vi "Subscribe (Async).vi"(9 "Topic":string, 10 "error in (no error)":errorcluster, 11 "WAMP Client in":refnum<class "WAMP Client.lvclass">) -> (1 "Request Result Event":refnum<user-event>, 2 "error out":errorcluster, 3 "WAMP Client out":refnum<class "WAMP Client.lvclass">)   [LabVIEW 2020, in "wamplv.lvlib" / "WAMP Client.lvclass"]
uses:
  <userlib>/wamplv/WAMP Client/WAMP Client.lvclass
  <userlib>/wamplv/WAMP Client/TypeDef/Subscribe Result.ctl
  <userlib>/wamplv/WAMP Client/TypeDef/Event Payload.ctl
  <userlib>/wamplv/WAMP Client/TypeDef/SUBSCRIBE Request Data.ctl
  <userlib>/wamplv/WAMP Client/TypeDef/Internal Message Type.ctl
  <userlib>/wamplv/WAMP Client/WAMP Client.lvclass/WAMP Client.ctl
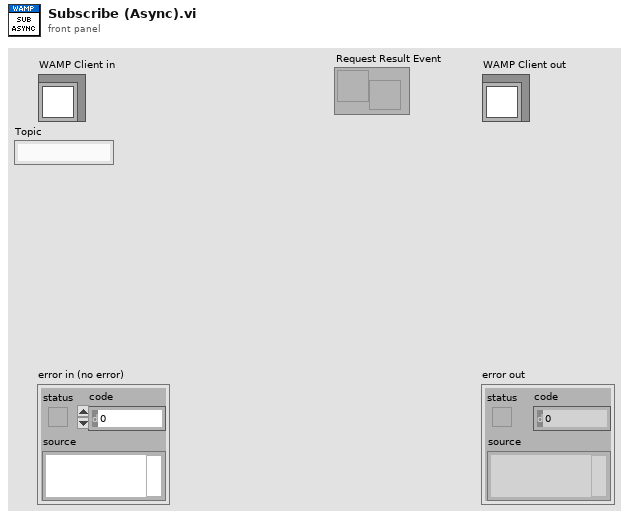
[diagram p1: front panel]
types:
  T1 = typedef "wamplv.lvlib/WAMP Client.lvclass/Internal Message Type.ctl" = enum16{"Subscribe", "Handle Subscribed", "Handle Event", "Unsubscribe", "Handle Unsubscribed", "Publish", "Handled Published", "Goodbye", "Handle Goodbye", "Call", "Handle Result", "Register", "Handle Registered", "Unregister", "Handle Unregistered", "Handle Invocation", "Yield"}
  T2 = typedef "wamplv.lvlib/WAMP Client.lvclass/Subscribe Result.ctl" = cluster{"Success?":bool, "Error":errorcluster, "Publication Received Event":refnum<user-event>}
  T3 = typedef "wamplv.lvlib/WAMP Client.lvclass/SUBSCRIBE Request Data.ctl" = cluster{"Topic":string, "Subscribe Response Received Event":refnum<user-event>}
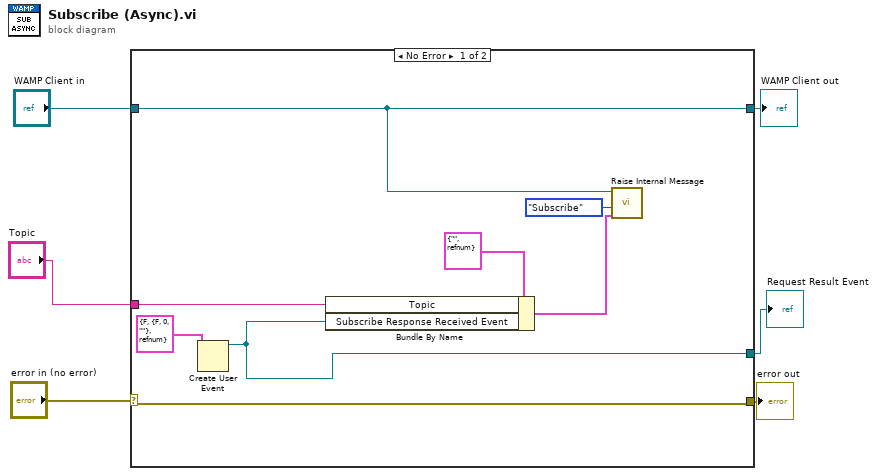
[diagram p0: block diagram]
diagram:
  n1 = case shown="No Error" "error in (no error)" {
    selector: "error in (no error)" -> [w14 w16]
    tunnel: [w14 w16] -> w5
    tunnel: [w13 w15] -> w3
    tunnel: "WAMP Client in" -> [w13 w15]
    tunnel: [w9 _] -> w2
    tunnel: "Topic" -> [w8 _]
    frame No Error {
      n2 = Create User Event(user event datatype=T2 {"Success?"=FALSE, "Error"={"status"=FALSE, "code"=0, "source"=""}, "Publication Received Event"=refnum} ("Subcsribe Result")) -> (user event=w9:refnum<user-event>)  [unwired: 1 in, 1 out]
      n3 = Bundle By Name(cluster=T3 {"Topic"="", "Subscribe Response Received Event"=refnum} ("Cluster"), "Topic"=w8, "Subscribe Response Received Event"=w9) -> (w10:T3)
      n4 = call-dynamic "Raise Internal Message.vi"("Variant"=w10, "Internal Message Type"=Internal_Message_Type."Subscribe", "WAMP Client in"=w13) -> ()  [unwired: 7 in, 2 out]
    }
    frame Error {
    }
  }
  "error out" <- w5
  "WAMP Client out" <- w3
  "Request Result Event" <- w2
